vi "SHA3-224 File Checksum.vi"(8 "error in":errorcluster, 11 "path":path) -> (0 "error out":errorcluster, 3 "digest":string)   [LabVIEW 2020, in "NI_Message Digest API.lvlib"]
doc: "Computes the message digest on the contents of a file. You must manually select the polymorphic instance you want to use."
uses:
  <vilib>/security/Message Digest/API/NI_Message Digest API.lvlib
  <vilib>/security/Message Digest/SHA-3/NI_SHA-3.lvclass/NI_SHA-3.ctl
  07e2d62d-d65e-48d1-912a-6d9031207283.vi
  07e2d62d-d65e-48d1-912a-6d9031207283.vi/9e5ab6c0-a93c-3fe1-04ae-efdc2201ed3f.vi
  <vilib>/security/Message Digest/SHA-3/Get Block Size.vi
  <vilib>/security/Message Digest/SHA-3/Get Block Size.vi/eb1e6525-3e01-40a8-a5c2-e849aaf68d04.vi
  <vilib>/security/Message Digest/SHA-3/Get Block Size.vi/eb1e6525-3e01-40a8-a5c2-e849aaf68d04.vi/00efce51-7697-47ef-971b-245e50795e7f.vi
  <vilib>/security/Message Digest/SHA-3/subVIs/Get Capacity.vi
  <vilib>/security/Message Digest/SHA-3/subVIs/Get Word Type.vi
  <vilib>/security/Message Digest/SHA-3/Reset.vi
  <vilib>/security/Message Digest/SHA-3/Append Block.vi
  <vilib>/security/Message Digest/SHA-3/Pad.vi
  <vilib>/security/Message Digest/SHA-3/Get Digest.vi
  <vilib>/security/Message Digest/SHA-3/NI_SHA-3.lvclass
  <vilib>/Bit Manipulation/NI_Bit Manipulation.lvlib
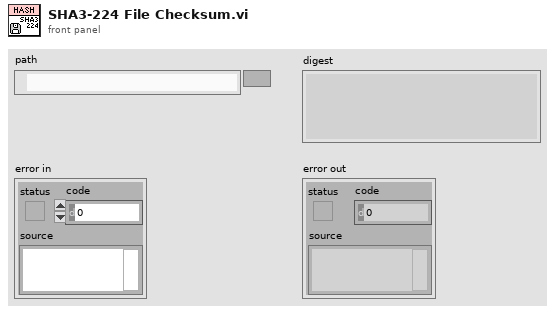
[diagram p1: front panel]
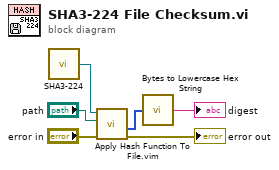
[diagram p0: block diagram]
diagram:
  n1 = call <vilib>:"SHA3-224.vi"() -> ("Hash Function out"=w2:refnum<class "NI_SHA-3.lvclass">)
  n2 = call "Apply Hash Function To File.vim"("error in"="error in", "path"="path", "Hash Function in (SHA-256)"=w2) -> ("error out"=→"error out":errorcluster, "digest"=w1:u8[])  [unwired: 6 in, 1 out]
  n3 = call <vilib>:"Bytes to Lowercase Hex String.vi"("bytes"=w1) -> ("hex string"=→"digest":string)
